vi "Queue_Buffer.vi"() -> ()   [LabVIEW 2020]
panel:
  out "Waveform Chart":dbl(graph)
  in  "stop":bool
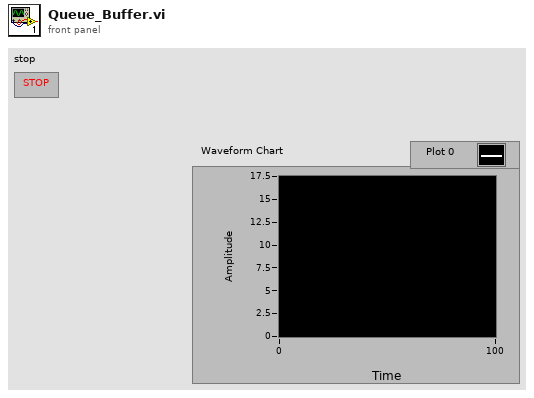
[diagram p1: front panel]
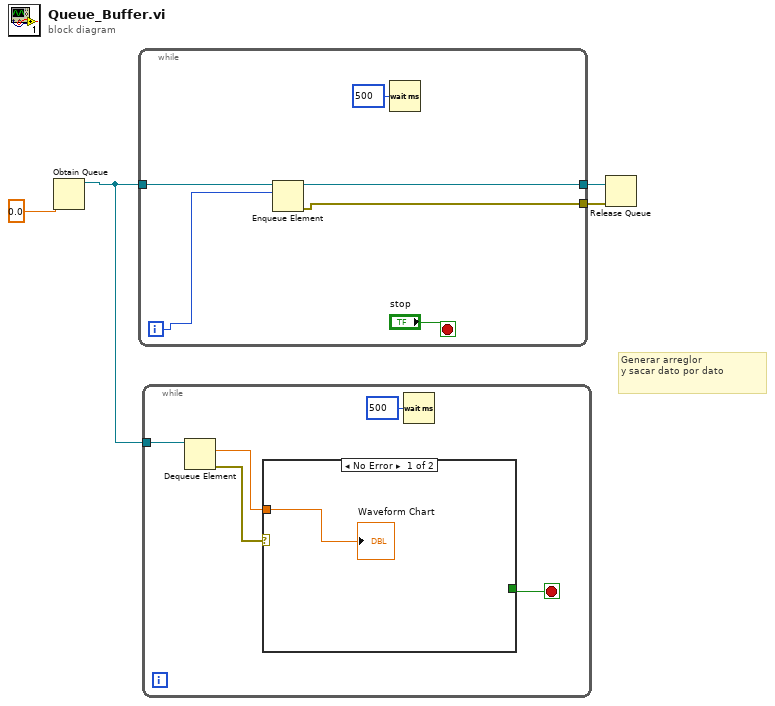
[diagram p0: block diagram]
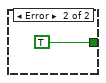
[diagram p2: hidden frame]
diagram:
  # "Generar arreglor \ny sacar dato por dato"
  n1 = Obtain Queue(element data type=0.0) -> (queue out=w3:refnum<queue>)  [unwired: 4 in, 2 out]
  n2 = while {
    tunnel: w3 -> [w10]
    tunnel: [w9] -> w2
    tunnel: [w5] -> w1
    i -> [w7]
    stop <- "stop" stop-if-true
    n3 = Enqueue Element(queue=w10, element=w7) -> (queue out=w9:refnum<queue>, error out=w5:errorcluster)  [unwired: 2 in, 1 out]
    n4 = Wait (ms)(milliseconds to wait=u32 500) -> ()  [unwired: 1 out]
  }
  n5 = while {
    tunnel: w3 -> [w15]
    stop <- w12 stop-if-true
    n6 = Dequeue Element(queue=w15) -> (element=w11:dbl, error out=w13:errorcluster)  [unwired: 2 in, 2 out]
    n7 = case shown="No Error" w13 {
      tunnel: [_ TRUE] -> w12
      tunnel: w11 -> [w16 _]
      frame No Error {
        "Waveform Chart" <- w16
      }
      frame Error {
      }
    }
    n8 = Wait (ms)(milliseconds to wait=u32 500) -> ()  [unwired: 1 out]
  }
  n9 = Release Queue(queue=w2, error in (no error)=w1) -> ()  [unwired: 1 in, 3 out]
